vi "update_attrs.vi"(8 "error in (no error)":errorcluster, 10 "Nested Enqueuers Map":T1(c390), 11 "DAQ Voltage in":refnum<class "DAQ Voltage.lvclass">) -> (0 "error out":errorcluster, 3 "DAQ Voltage out":refnum<class "DAQ Voltage.lvclass">)   [LabVIEW 2025, in "DAQ Voltage.lvlib" / "DAQ Voltage.lvclass"]
uses:
  DAQ Voltage.lvclass
  <vilib>/ActorFramework/Message Enqueuer/Message Enqueuer.lvclass
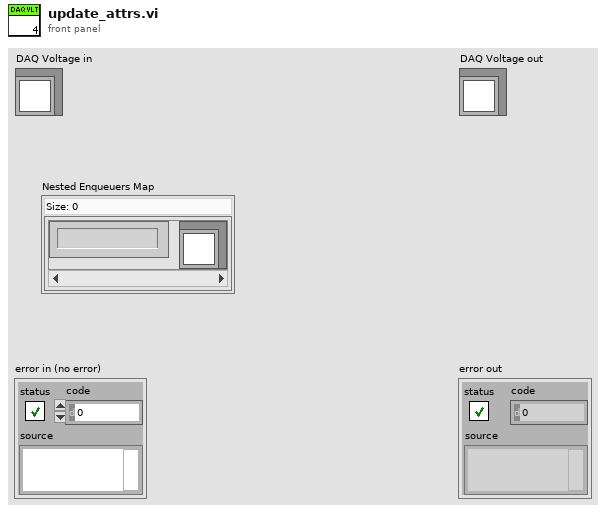
[diagram p1: front panel]
types:
  T1 = map{string, refnum<class "Message Enqueuer.lvclass">}
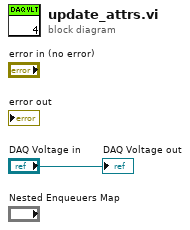
[diagram p0: block diagram]
diagram:
  "DAQ Voltage out" <- "DAQ Voltage in"
